vi "Read Iterator Decryption.vi"(11 "Circular Buffer in":refnum<class "Circular Buffer.lvclass">) -> (2 "Decryption":i64, 3 "Circular Buffer out":refnum<class "Circular Buffer.lvclass">)   [LabVIEW 2021, in "d20.lvlib" / "Circular Buffer.lvclass"]
uses:
  Circular Buffer.lvclass
  Circular Buffer.lvclass/Circular Buffer.ctl
  Node/Node.lvclass
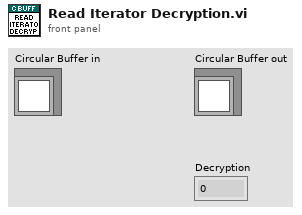
[diagram p1: front panel]
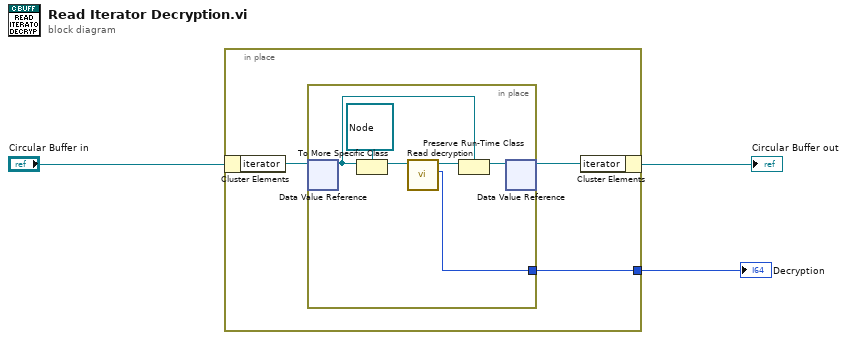
[diagram p0: block diagram]
diagram:
  n1 = in-place {
    in-place-border: [w5] -> w1
    n2 = in-place-cluster #1("Circular Buffer in") -> ("iterator"=w6:refnum<data-value>)
    n3 = in-place {
      in-place-border: [w9] -> w5
      n4 = in-place-dvr #2(w6) -> (w7:refnum<class>)  [unwired: 1 out]
      n5 = To More Specific Class(target class=refnum<class "Node.lvclass"> refnum ("d20.lvlib:Node.lvclass"), reference=w7) -> (specific class reference=w11:refnum<class "Node.lvclass">)  [unwired: 1 in, 1 out]
      n6 = call "Read decryption.vi"("Node in"=w11) -> ("decryption"=w9:i64, "Node out"=w10:refnum<class "Node.lvclass">)  [unwired: 9 in]
      n7 = Preserve Run-Time Class(object in=w10, 2:w7) -> (object out=w8:refnum<class>)  [unwired: 1 in, 1 out]
      n8 = in-place-dvr #2(w8) -> (w4:refnum<data-value>)  [unwired: 1 out]
    }
    n9 = in-place-cluster #1("iterator"=w4) -> (→"Circular Buffer out":refnum<class "Circular Buffer.lvclass">)
  }
  "Decryption" <- w1
